vi "Get DI State.vi"(8 "error in (no error)":errorcluster, 10 "DI IOName":string, 11 "DAQ":refnum<class "DAQ.lvclass">) -> (0 "error out":errorcluster, 1 "Timestamp (DBL)":dbl, 2 "State":bool, 3 "DAQ":refnum<class "DAQ.lvclass">, 5 "Time Stamp":timestamp)   [LabVIEW 2017, in "DAQ.lvclass"]
doc: "Developed by Kevin Thompson\nkevin@thompsonengineering.net\n\nCopyright 2018-2020\nThompson Engineering, LLC"
uses:
  DAQ.lvclass
  Process/ProcessSupport/TD DaqThread--enum.ctl
  DAQ.lvclass/DAQ.ctl
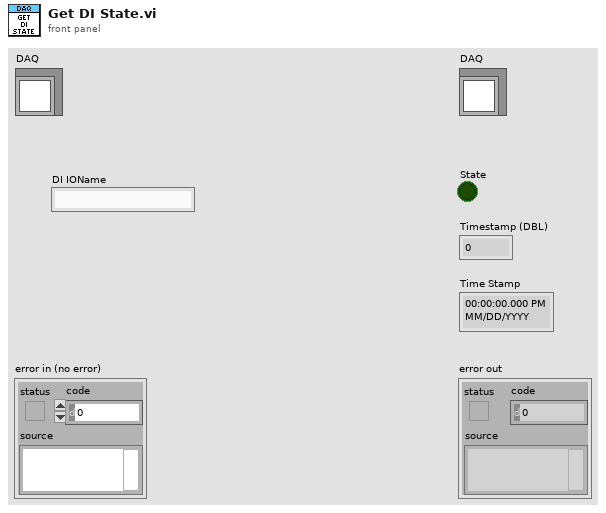
[diagram p1: front panel]
types:
  T1 = typedef "DAQ.lvclass/TD DaqThread--enum.ctl" = enum16{"AI", "DI"}
  T2 = typedef "TD Dynamic CVT DVR--ref.ctl" = refnum<data-value>
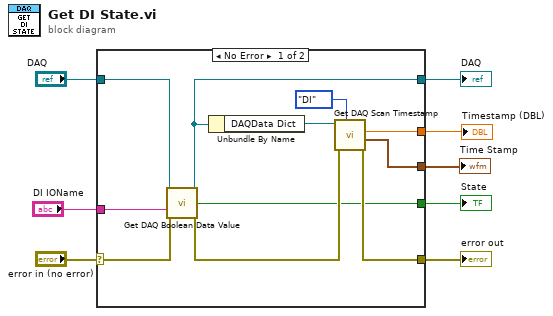
[diagram p0: block diagram]
diagram:
  n1 = case shown="No Error" "error in (no error)" {
    selector: "error in (no error)" -> [w19 w21]
    tunnel: [w14 w21] -> w7
    tunnel: [w17 w20] -> w5
    tunnel: "DAQ" -> [w18 w20]
    tunnel: "DI IOName" -> [w9 _]
    tunnel: [w12 _] -> w2
    tunnel: [w11 _] -> w3
    tunnel: [w10 _] -> w1
    frame No Error {
      n2 = call "Get DAQ Boolean Data Value.vi"("DAQ"=w18, "Name"=w9, "error in (no error)"=w19) -> ("DAQ"=w17:refnum<class "DAQ.lvclass">, "Value"=w10:bool, "error out"=w15:errorcluster)  [unwired: 10 in]
      n3 = Unbundle By Name(w17) -> ("DAQData Dict"=w16:T2)
      n4 = call "Get DAQ Scan Timestamp.vi"("Daq Thread"=TD_DaqThread--enum."DI", "error in (no error)"=w15, "DaqData dCVT"=w16) -> ("error out"=w14:errorcluster, "Time Stamp"=w11:timestamp, "Timestamp (DBL)"=w12:dbl)  [unwired: 5 in, 1 out]
    }
    frame Error {
    }
  }
  "error out" <- w7
  "DAQ" <- w5
  "State" <- w1
  "Time Stamp" <- w3
  "Timestamp (DBL)" <- w2
